vi "Log writer.vi"(10 "reference":refnum<vi>, 11 "string":string) -> ()   [LabVIEW 2016]
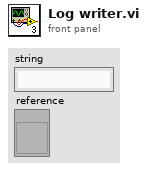
[diagram p1: front panel]
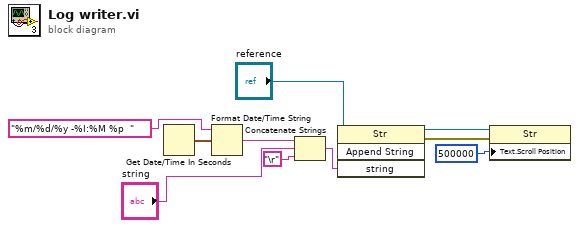
[diagram p0: block diagram]
diagram:
  n1 = Get Date/Time In Seconds() -> (seconds since 1Jan1904=w7:timestamp)
  n2 = Format Date/Time String(time format string (%c)="%m/%d/%y -%I:%M %p  ", seconds (now)=w7) -> (date/time string=w6:string)  [unwired: 1 in]
  n3 = Concatenate Strings(w6, "string", "\r") -> (w10:string)
  n4 = invoke on="Invoke Node" class="Str" method="Append String"(reference="reference", "string"=w10) -> (reference out=w1:refnum<vi>, error out=w4:errorcluster)  [unwired: 2 in, 2 out]
  n5 = property on="Property Node" class="Str"(reference=w1, error in=w4, "Text.Scroll Position"=u32 500000) -> ()  [unwired: 2 out]
